vi "ReadARINCFIFO.vi"(8 "error in":errorcluster, 11 "Refnum in":T1) -> (0 "error out":errorcluster, 3 "Data":u32[](array[numeric]))   [LabVIEW 2018, in "ARINC.lvlib"]
uses:
  ARINC.lvlib
  FPGA/Chassis3FPGARef.ctl
  <vilib>/Utility/error.llb/Error Cluster From Error Code.vi
  <vilib>/rvi/errors/niLvFpgaAdjustHostInterfaceError.vi
  <vilib>/rvi/interface/nirviMethod/nirviMethod.xnode
  <vilib>/FPGAPlugInAG/Dynamic/niLvFpga_ReadFifo_Dynamic.vi
  <vilib>/rvi/errors/niLvFpgaMergeErrorWithErrorCode.vi
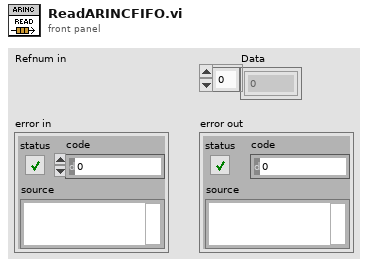
[diagram p1: front panel]
types:
  T1 = typedef "Chassis3FPGARef.ctl" = refnum<k20>
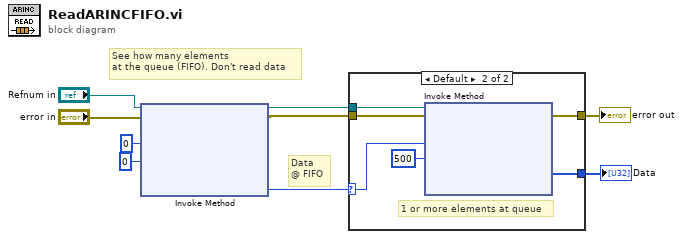
[diagram p0: block diagram]
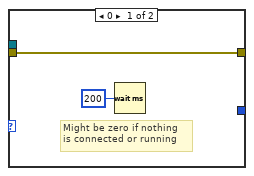
[diagram p2: hidden frame]
diagram:
  # "Data\n@ FIFO"
  # "See how many elements \nat the queue (FIFO). Don't read data"
  n1 = xnode "Invoke Method"("FPGA VI Reference In"="Refnum in", "error in"="error in", "Number of Elements"=u32 0, "Timeout (ms)"=0) -> ("FPGA VI Reference Out"=w4:T1, "error out"=w5:errorcluster, "Elements Remaining"=w1:u32)  [unwired: 1 out]
  n2 = case shown="Default" w1 {
    selector: w1 -> [_ w12]
    tunnel: [_ w17] -> w9
    tunnel: [w11 w16] -> w8
    tunnel: w5 -> [w11 w14]
    tunnel: w4 -> [_ w13]
    frame 0 {
      # "Might be zero if nothing\nis connected or running"
      n3 = Wait (ms)(milliseconds to wait=u32 200) -> ()  [unwired: 1 out]
    }
    frame Default {
      # "1 or more elements at queue"
      n4 = xnode "Invoke Method"("FPGA VI Reference In"=w13, "error in"=w14, "Number of Elements"=w12, "Timeout (ms)"=500) -> ("error out"=w16:errorcluster, "Data"=w17:u32[])  [unwired: 2 out]
    }
  }
  "Data" <- w9
  "error out" <- w8
